vi "pattern_request_TCP.vi"(1 "data in":string="bal bla bla") -> (0 "data out":u8[][](array[numeric]))   [LabVIEW 2011]
panel:
  out "error out":errorcluster
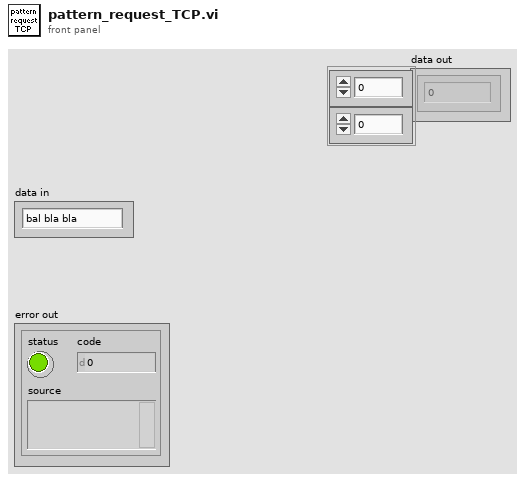
[diagram p1: front panel]
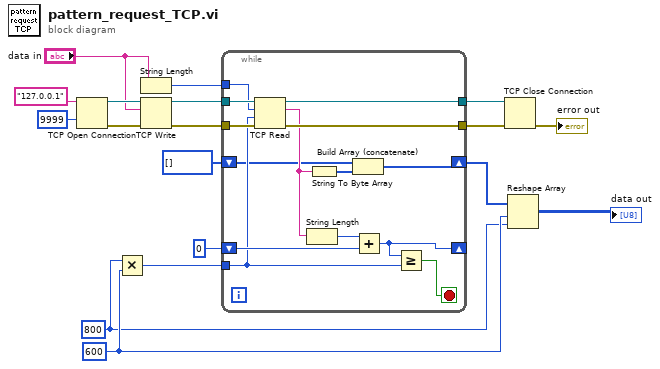
[diagram p0: block diagram]
diagram:
  w3 = 600 ("timeout ms (25000)")
  w2 = 800 ("timeout ms (25000)")
  n1 = TCP Open Connection(address="127.0.0.1", remote port or service name=u16 9999) -> (connection ID=w16:refnum<k5>, error out=w15:errorcluster)  [unwired: 3 in]
  n2 = Multiply(x=w2, y=w3) -> (x*y=w8:i32)
  n3 = String Length(string="data in") -> (length=w9:i32)
  n4 = TCP Write(connection ID=w16, data in="data in", error in (no error)=w15) -> (connection ID out=w11:refnum<k5>, error out=w14:errorcluster)  [unwired: 1 in, 1 out]
  n5 = while {
    tunnel: w14 -> [w32]
    tunnel: [w31] -> w13
    tunnel: [w30] -> w12
    tunnel: w11 -> [w29]
    tunnel: w9 -> [w28]
    tunnel: w8 -> [w24]
    shift-right: [w25] -> _
    shift-left: 0 ("timeout ms (25000)") -> [w26]
    shift-right: [w19] -> w4
    shift-left: u8[] [] -> [w20]
    stop <- w23 stop-if-true
    n6 = TCP Read(connection ID=w29, bytes to read=w28, error in (no error)=w32, 9:w24) -> (connection ID out=w30:refnum<k5>, data out=w22:string, error out=w31:errorcluster)  [unwired: 1 in]
    n7 = String Length(string=w22) -> (length=w27:i32)
    n8 = String To Byte Array(string=w22) -> (unsigned byte array=w21:u8[])
    n9 = Build Array (concatenate)(w20, w21) -> (w19:u8[])
    n10 = Add(x=w27, y=w26) -> (x+y=w25:i32)
    n11 = Greater Or Equal?(x=w25, y=w24) -> (x >= y?=w23:bool)
  }
  n12 = TCP Close Connection(connection ID=w12, error in (no error)=w13) -> (error out=→"error out":errorcluster)  [unwired: 1 in, 1 out]
  n13 = Reshape Array(w4, w3, w2) -> (→"data out":u8[][])
